vi "SplitLR.vi"(3 "Vision Targets":dbl[][](array[numeric])) -> (0 "Right":dbl[](array[numeric]), 1 "Left":dbl[](array[numeric]))   [LabVIEW 2016]
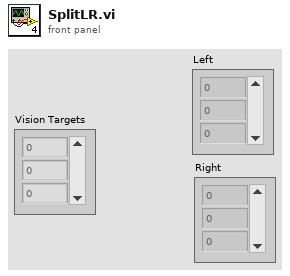
[diagram p1: front panel]
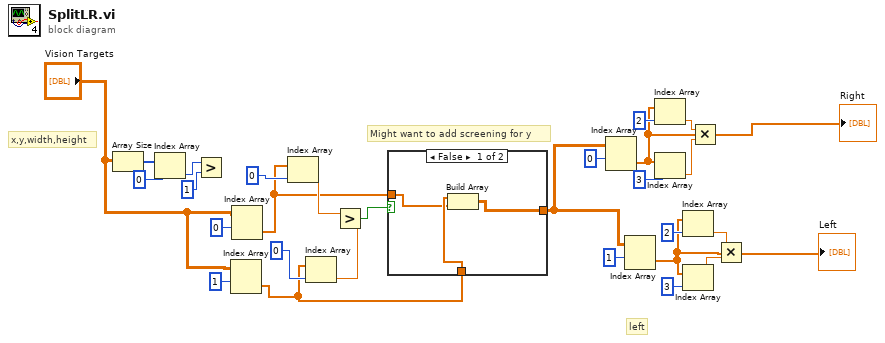
[diagram p0: block diagram]
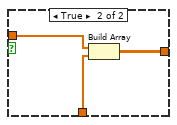
[diagram p2: hidden frame]
diagram:
  # "left"
  # "Might want to add screening for y"
  # "x,y,width,height"
  n1 = Array Size(array="Vision Targets") -> (size(s)=w27:i32[])
  n2 = Index Array(array=w27, index=0) -> (element=w25:i32)
  n3 = Greater?(x=w25, y=1) -> ()  [unwired: 1 out]
  n4 = Index Array(array="Vision Targets", index (row)=1) -> (element=w16:dbl[])  [unwired: 1 in]
  n5 = Index Array(array="Vision Targets", index (row)=0) -> (element=w17:dbl[])  [unwired: 1 in]
  n6 = Index Array(array=w17, index=0) -> (element=w19:dbl)
  n7 = Index Array(array=w16, index=0) -> (element=w18:dbl)
  n8 = Greater?(x=w19, y=w18) -> (0:w15:bool)
  n9 = case shown="False" w15 {
    tunnel: w17 -> [w29 w33]
    tunnel: w16 -> [w30 w32]
    tunnel: [w28 w31] -> w12
    frame False {
      n10 = Build Array(w30, w29) -> (w28:dbl[][])
    }
    frame True {
      n11 = Build Array(w33, w32) -> (w31:dbl[][])
    }
  }
  n12 = Index Array(array=w12, index (row)=0) -> (element=w2:dbl[])  [unwired: 1 in]
  "Right" <- w2
  n13 = Index Array(array=w12, index (row)=1) -> (element=w1:dbl[])  [unwired: 1 in]
  "Left" <- w1
  n14 = Index Array(array=w2, index=2) -> (element=w7:dbl)
  n15 = Index Array(array=w2, index=3) -> (element=w6:dbl)
  n16 = Index Array(array=w1, index=2) -> (element=w5:dbl)
  n17 = Index Array(array=w1, index=3) -> (element=w4:dbl)
  n18 = Multiply(x=w7, y=w6) -> ()  [unwired: 1 out]
  n19 = Multiply(x=w5, y=w4) -> ()  [unwired: 1 out]
